vi "Arduino Stepper Driver XY for Dual Etalon.vi"() -> ()   [LabVIEW 2013]
uses:
  Custom Controls/SV Hosts.ctl
  <vilib>/Instr/_visa.llb/VISA Flush IO Buffer Mask.ctl
  <vilib>/Utility/error.llb/DialogType.ctl
  <vilib>/Instr/_visa.llb/VISA Configure Serial Port (Instr).vi
panel:
  out "Motor Ready":bool
  in  "Motor COM Port":refnum<visa-resource-name>="COM4"
  in  "Shared Variable Target":T1=enum."RILIS-VM"
  in  "Horizontal driver setpoint":i32
  in  "Vertical driver setpoint":i32
  out "Out of Range!":bool
  out "number of errors":i32
  out "Vertical driver position":i32
  out "Horizontal driver position":i32
  out "ERROR":bool
  out "loop timer":u32
  in  "Reset Driver to 0":bool
  out "loop counter":i32
  in  "stop":bool
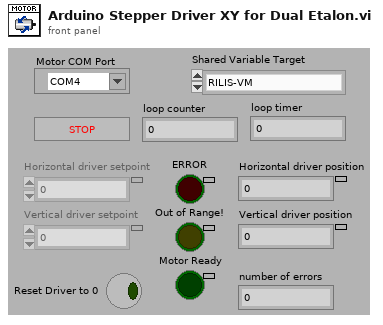
[diagram p1: front panel]
types:
  T1 = typedef "SV Hosts.ctl" = enum16{"LocalHost", "RILIS-VM", "RILIS-VM backup", "RILIS-SERVER"}
  T2 = typedef "VISA Flush IO Buffer Mask.ctl" = u16
  T3 = typedef "DialogType.ctl" = u16
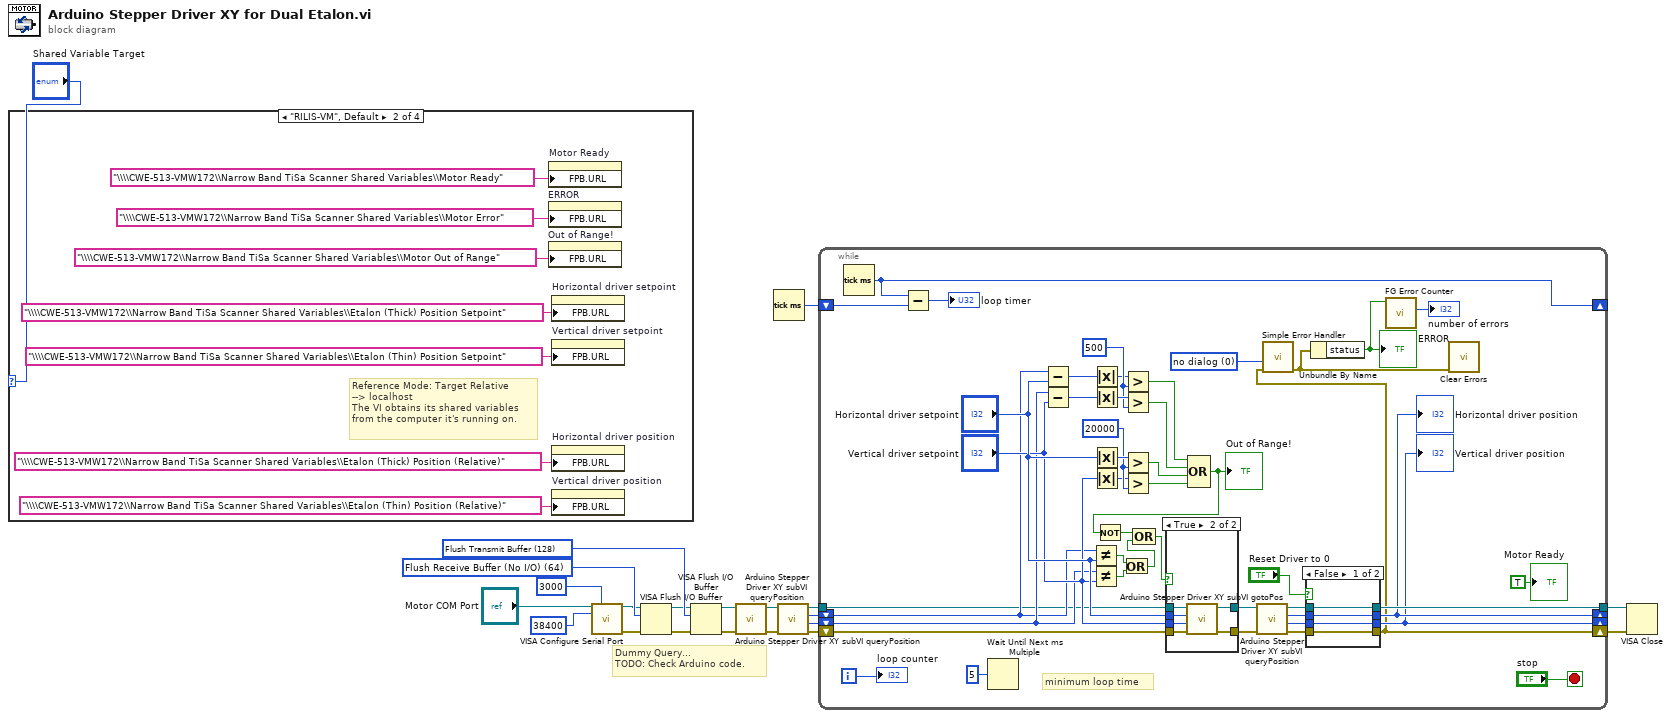
[diagram p0: block diagram]
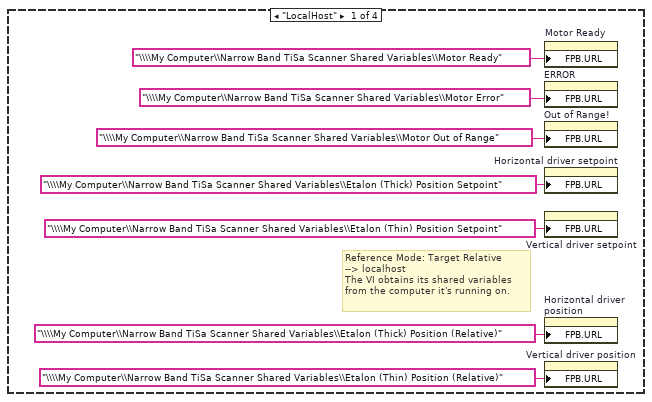
[diagram p2: hidden frame]
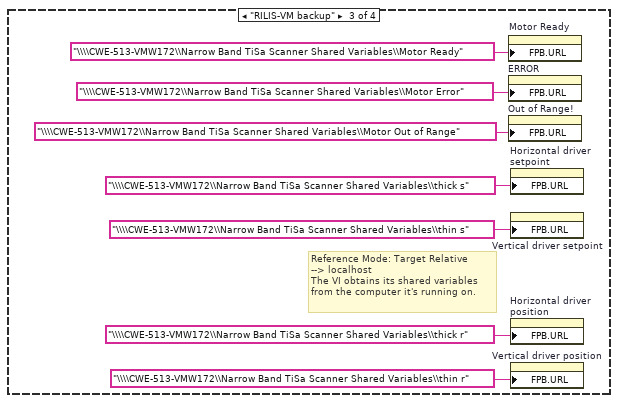
[diagram p3: hidden frame]
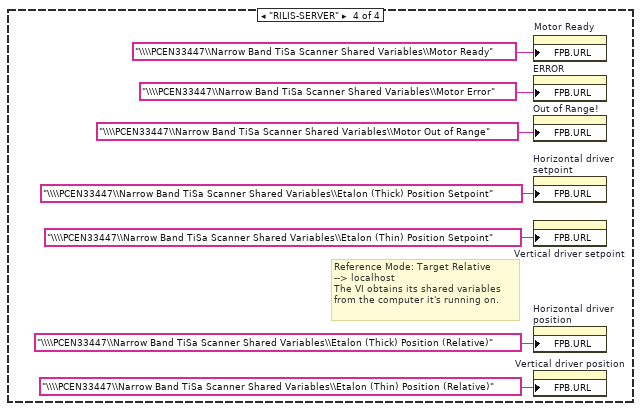
[diagram p4: hidden frame]
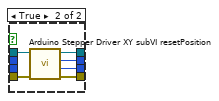
[diagram p6: hidden frame]
diagram:
  w9 = T2 64 items=["Flush Receive Buffer"=16, "Write Transmit Buffer to Device"=32, "Flush Receive Buffer (No I/O)"=64, "Flush Transmit Buffer"=128] ("Mask")
  w10 = T2 128 items=["Flush Receive Buffer"=16, "Write Transmit Buffer to Device"=32, "Flush Receive Buffer (No I/O)"=64, "Flush Transmit Buffer"=128] ("Mask")
  # "Dummy Query...\nTODO: Check Arduino code."
  n1 = case shown="\"RILIS-VM\", Default" "Shared Variable Target" {
    frame "LocalHost" {
      # "Reference Mode: Target Relative\n--> localhost\nThe VI obtains its shared variables\nfrom the computer it's running on."
      n2 = property on="Motor Ready" class="Bool (strict)"("FPB.URL"="\\\\My Computer\\Narrow Band TiSa Scanner Shared Variables\\Motor Ready" ("Data Binding:Path")) -> ()  [unwired: 2 in, 2 out]
      n3 = property on="ERROR" class="Bool (strict)"("FPB.URL"="\\\\My Computer\\Narrow Band TiSa Scanner Shared Variables\\Motor Error" ("Data Binding:Path")) -> ()  [unwired: 2 in, 2 out]
      n4 = property on="Out of Range!" class="Bool (strict)"("FPB.URL"="\\\\My Computer\\Narrow Band TiSa Scanner Shared Variables\\Motor Out of Range" ("Data Binding:Path")) -> ()  [unwired: 2 in, 2 out]
      n5 = property on="Horizontal driver setpoint" class="DigNum (strict)"("FPB.URL"="\\\\My Computer\\Narrow Band TiSa Scanner Shared Variables\\Etalon (Thick) Position Setpoint" ("Data Binding:Path")) -> ()  [unwired: 2 in, 2 out]
      n6 = property on="Vertical driver setpoint" class="DigNum (strict)"("FPB.URL"="\\\\My Computer\\Narrow Band TiSa Scanner Shared Variables\\Etalon (Thin) Position Setpoint" ("Data Binding:Path")) -> ()  [unwired: 2 in, 2 out]
      n7 = property on="Horizontal driver position" class="DigNum (strict)"("FPB.URL"="\\\\My Computer\\Narrow Band TiSa Scanner Shared Variables\\Etalon (Thick) Position (Relative)" ("Data Binding:Path")) -> ()  [unwired: 2 in, 2 out]
      n8 = property on="Vertical driver position" class="DigNum (strict)"("FPB.URL"="\\\\My Computer\\Narrow Band TiSa Scanner Shared Variables\\Etalon (Thin) Position (Relative)" ("Data Binding:Path")) -> ()  [unwired: 2 in, 2 out]
    }
    frame "RILIS-VM", Default {
      # "Reference Mode: Target Relative\n--> localhost\nThe VI obtains its shared variables\nfrom the computer it's running on."
      n9 = property on="Motor Ready" class="Bool (strict)"("FPB.URL"="\\\\CWE-513-VMW172\\Narrow Band TiSa Scanner Shared Variables\\Motor Ready" ("Data Binding:Path")) -> ()  [unwired: 2 in, 2 out]
      n10 = property on="ERROR" class="Bool (strict)"("FPB.URL"="\\\\CWE-513-VMW172\\Narrow Band TiSa Scanner Shared Variables\\Motor Error" ("Data Binding:Path")) -> ()  [unwired: 2 in, 2 out]
      n11 = property on="Out of Range!" class="Bool (strict)"("FPB.URL"="\\\\CWE-513-VMW172\\Narrow Band TiSa Scanner Shared Variables\\Motor Out of Range" ("Data Binding:Path")) -> ()  [unwired: 2 in, 2 out]
      n12 = property on="Horizontal driver setpoint" class="DigNum (strict)"("FPB.URL"="\\\\CWE-513-VMW172\\Narrow Band TiSa Scanner Shared Variables\\Etalon (Thick) Position Setpoint" ("Data Binding:Path")) -> ()  [unwired: 2 in, 2 out]
      n13 = property on="Vertical driver setpoint" class="DigNum (strict)"("FPB.URL"="\\\\CWE-513-VMW172\\Narrow Band TiSa Scanner Shared Variables\\Etalon (Thin) Position Setpoint" ("Data Binding:Path")) -> ()  [unwired: 2 in, 2 out]
      n14 = property on="Horizontal driver position" class="DigNum (strict)"("FPB.URL"="\\\\CWE-513-VMW172\\Narrow Band TiSa Scanner Shared Variables\\Etalon (Thick) Position (Relative)" ("Data Binding:Path")) -> ()  [unwired: 2 in, 2 out]
      n15 = property on="Vertical driver position" class="DigNum (strict)"("FPB.URL"="\\\\CWE-513-VMW172\\Narrow Band TiSa Scanner Shared Variables\\Etalon (Thin) Position (Relative)" ("Data Binding:Path")) -> ()  [unwired: 2 in, 2 out]
    }
    frame "RILIS-VM backup" {
      # "Reference Mode: Target Relative\n--> localhost\nThe VI obtains its shared variables\nfrom the computer it's running on."
      n16 = property on="Motor Ready" class="Bool (strict)"("FPB.URL"="\\\\CWE-513-VMW172\\Narrow Band TiSa Scanner Shared Variables\\Motor Ready" ("Data Binding:Path")) -> ()  [unwired: 2 in, 2 out]
      n17 = property on="ERROR" class="Bool (strict)"("FPB.URL"="\\\\CWE-513-VMW172\\Narrow Band TiSa Scanner Shared Variables\\Motor Error" ("Data Binding:Path")) -> ()  [unwired: 2 in, 2 out]
      n18 = property on="Out of Range!" class="Bool (strict)"("FPB.URL"="\\\\CWE-513-VMW172\\Narrow Band TiSa Scanner Shared Variables\\Motor Out of Range" ("Data Binding:Path")) -> ()  [unwired: 2 in, 2 out]
      n19 = property on="Horizontal driver setpoint" class="DigNum (strict)"("FPB.URL"="\\\\CWE-513-VMW172\\Narrow Band TiSa Scanner Shared Variables\\thick s" ("Data Binding:Path")) -> ()  [unwired: 2 in, 2 out]
      n20 = property on="Vertical driver setpoint" class="DigNum (strict)"("FPB.URL"="\\\\CWE-513-VMW172\\Narrow Band TiSa Scanner Shared Variables\\thin s" ("Data Binding:Path")) -> ()  [unwired: 2 in, 2 out]
      n21 = property on="Horizontal driver position" class="DigNum (strict)"("FPB.URL"="\\\\CWE-513-VMW172\\Narrow Band TiSa Scanner Shared Variables\\thick r" ("Data Binding:Path")) -> ()  [unwired: 2 in, 2 out]
      n22 = property on="Vertical driver position" class="DigNum (strict)"("FPB.URL"="\\\\CWE-513-VMW172\\Narrow Band TiSa Scanner Shared Variables\\thin r" ("Data Binding:Path")) -> ()  [unwired: 2 in, 2 out]
    }
    frame "RILIS-SERVER" {
      # "Reference Mode: Target Relative\n--> localhost\nThe VI obtains its shared variables\nfrom the computer it's running on."
      n23 = property on="Motor Ready" class="Bool (strict)"("FPB.URL"="\\\\PCEN33447\\Narrow Band TiSa Scanner Shared Variables\\Motor Ready" ("Data Binding:Path")) -> ()  [unwired: 2 in, 2 out]
      n24 = property on="ERROR" class="Bool (strict)"("FPB.URL"="\\\\PCEN33447\\Narrow Band TiSa Scanner Shared Variables\\Motor Error" ("Data Binding:Path")) -> ()  [unwired: 2 in, 2 out]
      n25 = property on="Out of Range!" class="Bool (strict)"("FPB.URL"="\\\\PCEN33447\\Narrow Band TiSa Scanner Shared Variables\\Motor Out of Range" ("Data Binding:Path")) -> ()  [unwired: 2 in, 2 out]
      n26 = property on="Horizontal driver setpoint" class="DigNum (strict)"("FPB.URL"="\\\\PCEN33447\\Narrow Band TiSa Scanner Shared Variables\\Etalon (Thick) Position Setpoint" ("Data Binding:Path")) -> ()  [unwired: 2 in, 2 out]
      n27 = property on="Vertical driver setpoint" class="DigNum (strict)"("FPB.URL"="\\\\PCEN33447\\Narrow Band TiSa Scanner Shared Variables\\Etalon (Thin) Position Setpoint" ("Data Binding:Path")) -> ()  [unwired: 2 in, 2 out]
      n28 = property on="Horizontal driver position" class="DigNum (strict)"("FPB.URL"="\\\\PCEN33447\\Narrow Band TiSa Scanner Shared Variables\\Etalon (Thick) Position (Relative)" ("Data Binding:Path")) -> ()  [unwired: 2 in, 2 out]
      n29 = property on="Vertical driver position" class="DigNum (strict)"("FPB.URL"="\\\\PCEN33447\\Narrow Band TiSa Scanner Shared Variables\\Etalon (Thin) Position (Relative)" ("Data Binding:Path")) -> ()  [unwired: 2 in, 2 out]
    }
  }
  n30 = call-poly "VISA Configure Serial Port"("VISA resource name"="Motor COM Port", "timeout (10sec)"=u32 3000, "baud rate (9600)"=u32 38400) -> ("VISA resource name out"=w8:refnum<visa-resource-name>, "error out"=w7:errorcluster)  [unwired: 11 in]
  n31 = VISA Flush I/O Buffer(VISA resource name=w8, mask (16)=w9, error in (no error)=w7) -> (VISA resource name out=w5:refnum<visa-resource-name>, error out=w6:errorcluster)
  n32 = VISA Flush I/O Buffer(VISA resource name=w5, mask (16)=w10, error in (no error)=w6) -> (VISA resource name out=w18:refnum<visa-resource-name>, error out=w17:errorcluster)
  n33 = call "Arduino Stepper Driver XY subVI queryPosition.vi"("error in (no error)"=w17, "VISA resource name"=w18) -> ("error out"=w12:errorcluster, "VISA resource name out"=w13:refnum<visa-resource-name>)  [unwired: 6 in, 2 out]
  n34 = Tick Count (ms)() -> (millisecond timer value=w14:u32)
  n35 = call "Arduino Stepper Driver XY subVI queryPosition.vi"("error in (no error)"=w12, "VISA resource name"=w13) -> ("error out"=w4:errorcluster, "Vertical driver position"=w3:i32, "Horizontal driver position"=w2:i32, "VISA resource name out"=w11:refnum<visa-resource-name>)  [unwired: 6 in]
  n36 = while {
    tunnel: w11 -> [w51]
    shift-right: [w57] -> _
    shift-left: w2 -> [w52]
    shift-right: [w56] -> _
    shift-left: w3 -> [w53]
    tunnel: [w58] -> w16
    shift-right: [w84] -> _
    shift-left: w14 -> [w85]
    shift-right: [w55] -> w15
    shift-left: w4 -> [w54]
    i -> [w93]
    stop <- "stop" stop-if-true
    w68 = 500
    w76 = 20000
    w82 = T3 0 items=["no dialog", "OK message", "continue or stop message", "OK message + warnings", "continue/stop + warnings"] ("type of dialog (OK msg:1)")
    # "minimum loop time"
    n37 = Tick Count (ms)() -> (millisecond timer value=w84:u32)
    n38 = Subtract(x=w84, y=w85) -> (x-y=→"loop timer":u32)
    n39 = Wait Until Next ms Multiple(millisecond multiple=u32 5) -> ()  [unwired: 1 out]
    n40 = Subtract(x=w52, y="Horizontal driver setpoint") -> (x-y=w66:i32)
    n41 = Subtract(x=w53, y="Vertical driver setpoint") -> (x-y=w65:i32)
    n42 = Not Equal?(x=w52, y="Horizontal driver setpoint") -> (x != y?=w81:bool)
    n43 = Not Equal?(x=w53, y="Vertical driver setpoint") -> (x != y?=w80:bool)
    n44 = Absolute Value(x=w66) -> (abs(x)=w67:i32)
    n45 = Absolute Value(x=w65) -> (abs(x)=w69:i32)
    n46 = Absolute Value(x="Horizontal driver setpoint") -> (abs(x)=w77:i32)
    n47 = Absolute Value(x="Vertical driver setpoint") -> (abs(x)=w75:i32)
    n48 = Or(x=w81, y=w80) -> (x .or. y?=w72:bool)
    n49 = Greater?(x=w67, y=w68) -> (0:w64:bool)
    n50 = Greater?(x=w69, y=w68) -> (0:w63:bool)
    n51 = Greater?(x=w77, y=w76) -> (0:w74:bool)
    n52 = Greater?(x=w75, y=w76) -> (0:w73:bool)
    n53 = Compound Arithmetic op=OR(w64, w63, w74, w73) -> (w62:bool)
    "Out of Range!" <- w62
    n54 = Not(x=w62) -> (.not. x?=w70:bool)
    n55 = Compound Arithmetic op=OR(w70, w72) -> (w71:bool)
    n56 = case shown="True" w71 {
      tunnel: [w96 w103] -> w92
      tunnel: w51 -> [w97 w102]
      tunnel: w54 -> [w96 w101]
      tunnel: [w97 w100] -> w91
      tunnel: "Vertical driver setpoint" -> [_ w99]
      tunnel: "Horizontal driver setpoint" -> [_ w98]
      frame False {
      }
      frame True {
        n57 = call "Arduino Stepper Driver XY subVI gotoPos.vi"("error in (no error)"=w101, "Vertical Set Position"=w99, "Horizontal Set Position"=w98, "VISA resource name"=w102) -> ("error out"=w103:errorcluster, "VISA resource name out"=w100:refnum<visa-resource-name>)  [unwired: 6 in]
      }
    }
    n58 = call "Arduino Stepper Driver XY subVI queryPosition.vi"("error in (no error)"=w92, "VISA resource name"=w91) -> ("error out"=w89:errorcluster, "Vertical driver position"=w86:i32, "Horizontal driver position"=w87:i32, "VISA resource name out"=w90:refnum<visa-resource-name>)  [unwired: 6 in]
    n59 = case shown="False" "Reset Driver to 0" {
      tunnel: w90 -> [w107 w113]
      tunnel: w89 -> [w106 w112]
      tunnel: [w106 w111] -> w55
      tunnel: [w107 w110] -> w58
      tunnel: [w105 w109] -> w57
      tunnel: [w104 w108] -> w56
      tunnel: w87 -> [w105 _]
      tunnel: w86 -> [w104 _]
      frame False {
      }
      frame True {
        n60 = call "Arduino Stepper Driver XY subVI resetPosition.vi"("error in (no error)"=w112, "VISA resource name"=w113) -> ("error out"=w111:errorcluster, "Vertical driver position"=w108:i32, "Horizontal driver position"=w109:i32, "VISA resource name out"=w110:refnum<visa-resource-name>)  [unwired: 6 in]
      }
    }
    "Horizontal driver position" <- w57
    "Vertical driver position" <- w56
    n61 = call <vilib>:"Simple Error Handler.vi"("type of dialog (OK msg:1)"=w82, "error in (no error)"=w55) -> ("error out"=w78:errorcluster)  [unwired: 3 in, 4 out]
    n62 = Unbundle By Name(w78) -> ("status"=w61:bool)
    "ERROR" <- w61
    n63 = call "FG Error Counter.vi"("reset to 0"=w61) -> ("number of errors"=→"number of errors":i32)  [unwired: 10 in]
    n64 = call <vilib>:"Clear Errors.vi"("error in (no error)"=w78) -> ()  [unwired: 6 in, 1 out]
    "loop counter" <- w93
    "Motor Ready" <- TRUE
  }
  n65 = VISA Close(VISA resource name=w16, error in (no error)=w15) -> ()  [unwired: 1 out]
